vi "Plot Name.vi"(7 "error in":errorcluster, 10 "challenge":T1) -> (0 "error out":errorcluster, 3 "plot name":string)   [LabVIEW 2011]
uses:
  PID/Controls/Challenge.ctl
  Controls/Concentration Units.ctl
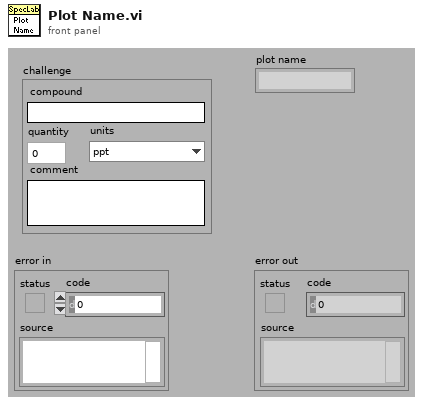
[diagram p1: front panel]
types:
  T1 = typedef "Challenge.ctl" = cluster{"compound":string, "quantity":dbl, "units":T2, "comment":string}
  T2 = typedef "Concentration Units.ctl" = enum16{"ppt", "ppb", "ppm"}
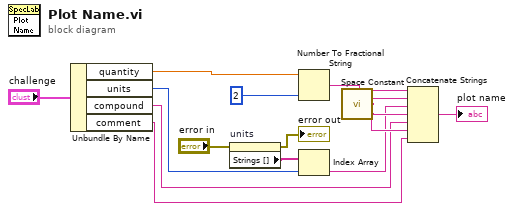
[diagram p0: block diagram]
diagram:
  n1 = Unbundle By Name("challenge") -> ("quantity"=w6:dbl, "units"=w8:T2, "compound"=w9:string, "comment"=w11:string)
  n2 = property on="units" class="Enum (strict)"(error in="error in") -> (error out=→"error out":errorcluster, "Strings []"=w4:string[])  [unwired: 1 in, 1 out]
  n3 = Number To Fractional String(number=w6, precision (6)=i16 2) -> (F-format string=w7:string)  [unwired: 2 in]
  n4 = Index Array(array=w4, index=w8) -> (element=w1:string)
  n5 = call <vilib>:"Space Constant.vi"() -> ("String"=w10:string)
  n6 = Concatenate Strings(w7, w10, w1, w10, w9, w10, w11) -> (→"plot name":string)
